vi "Setpoint.vi"(8 "error in (no error)":errorcluster, 10 "Setpoint [T]":dbl format="%.5f", 11 "PS Control Actor in":refnum<class "PS Control Actor.lvclass">) -> (0 "error out":errorcluster, 2 "Setpoint out":dbl, 3 "PS Control Actor out":refnum<class "PS Control Actor.lvclass">)   [LabVIEW 2025, in "PS Control Actor.lvlib" / "PS Control Actor.lvclass"]
doc: "Author: Scott Hannahs <sth@magnet.fsu.edu>\n\nThis software is licensed for use under the “MIT License\"\nCopyright (c) 2025 Scott Hannahs, sth@sth@magnet.sthnet.net\n\nPermission is hereby granted, free of charge, to any person obtaining a copy of this software and associated documentation files (the \"Software\"), to deal in the Software without restriction, including without limitation the rights to use, copy, modify, merge, publish, distribute, sublicense, and/or sell copies of the Software, and to permit persons to whom the Software is furnished to do so, subject to the following conditions: The above copyright notice and this permission notice shall be included in all copies or substantial portions of the Software.\n\nTHE SOFTWARE IS PROVIDED \"AS IS\", WITHOUT WARRANTY OF ANY KIND, EXPRESS OR IMPLIED, INCLUDING BUT NOT LIMITED TO THE WARRANTIES OF MERCHANTABILITY, FITNESS FOR A PARTICULAR PURPOSE AND NONINFRINGEMENT. IN NO EVENT SHALL THE AUTHORS OR COPYRIGHT HOLDERS BE LIABLE FOR ANY CLAIM, DAMAGES OR OTHER LIABILITY, WHETHER IN AN ACTION OF CONTRACT, TORT OR OTHERWISE, ARISING FROM, OUT OF OR IN CONNECTION WITH THE SOFTWARE OR THE USE OR OTHER DEALINGS IN THE SOFTWARE."
uses:
  PS Control Actor.lvclass
  PS Control Actor.lvclass/PS Control Actor.ctl
  PS Driver/PS Driver.lvclass
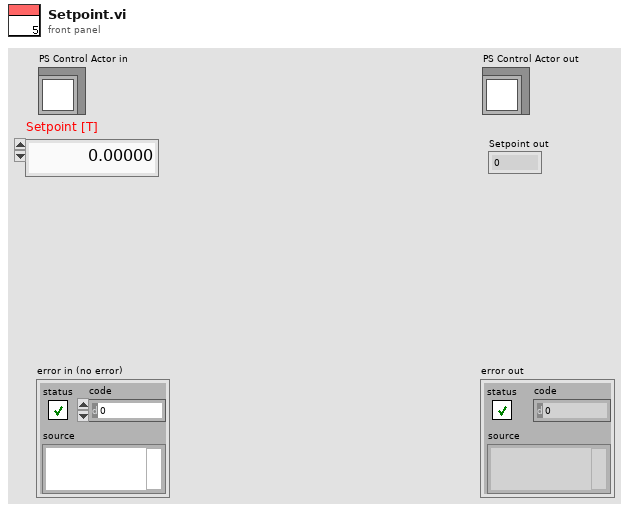
[diagram p1: front panel]
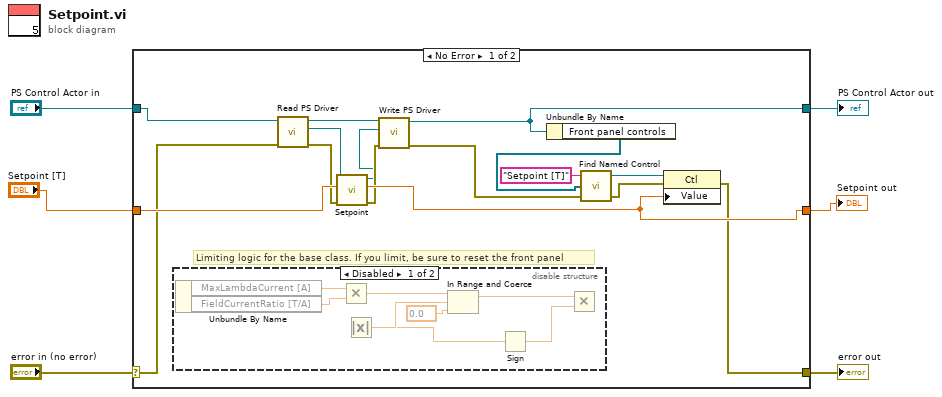
[diagram p0: block diagram]
diagram:
  n1 = case shown="No Error" "error in (no error)" {
    selector: "error in (no error)" -> [w9 w33]
    tunnel: [w16 w33] -> w5
    tunnel: [w13 w32] -> w3
    tunnel: "PS Control Actor in" -> [w15 w32]
    tunnel: "Setpoint [T]" -> [w22 w31]
    tunnel: [w17 w31] -> w1
    frame No Error {
      # "Limiting logic for the base class. If you limit, be sure to reset the front panel"
      n2 = disable-structure shown="Disabled" {
        frame Disabled {
          n3 = Unbundle By Name() -> ("MaxLambdaCurrent [A]"=w29:dbl, "FieldCurrentRatio [T/A]"=w28:dbl)  [unwired: 1 in]
          n4 = Multiply(x=w29, y=w28) -> (x*y=w30:dbl)
          n5 = Absolute Value() -> (x=w24:dbl, abs(x)=w27:dbl)
          n6 = In Range and Coerce(upper limit=w30, x=w27, lower limit=0.0) -> (coerced(x)=w25:dbl)  [unwired: 1 out]
          n7 = Sign(1:w24) -> (0:w23:dbl)
          n8 = Multiply(x=w25, y=w23) -> ()  [unwired: 1 out]
        }
        frame Enabled {
        }
      }
      n9 = call-dynamic "Read PS Driver.vi"("error in (no error)"=w9, "PS Control Actor in"=w15) -> ("error out"=w10:errorcluster, "PS Driver.lvlib:PS Driver.lvclass"=w8:refnum<class "PS Driver.lvclass">, "PS Control Actor out"=w14:refnum<class "PS Control Actor.lvclass">)  [unwired: 7 in]
      n10 = call-dynamic "Setpoint.vi"("error in (no error)"=w10, "Setpoint [A]"=w22, "PS Driver.lvlib:PS Driver.lvclass in"=w8) -> ("error out"=w11:errorcluster, "Setpoint out (A)"=w17:dbl, "PS Driver.lvlib:PS Driver.lvclass out"=w7:refnum<class "PS Driver.lvclass">)  [unwired: 6 in]
      n11 = call-dynamic "Write PS Driver.vi"("error in (no error)"=w11, "PS Driver.lvlib:PS Driver.lvclass"=w7, "PS Control Actor in"=w14) -> ("error out"=w12:errorcluster, "PS Control Actor out"=w13:refnum<class "PS Control Actor.lvclass">)  [unwired: 7 in]
      n12 = Unbundle By Name(w13) -> ("Front panel controls"=w19:refnum<vi>[])
      n13 = call "Find Named Control.vi"("error in"=w12, "All Controls"=w19, "Control Name"="Setpoint [T]") -> ("error out"=w21:errorcluster, "Ctl Refnum"=w18:refnum<vi>)  [unwired: 1 out]
      n14 = property class="Ctl"(reference=w18, error in=w21, "Value"=w17) -> (error out=w16:errorcluster)  [unwired: 1 out]
    }
    frame Error {
    }
  }
  "error out" <- w5
  "PS Control Actor out" <- w3
  "Setpoint out" <- w1
